vi "Write Micron Configuration.vi"(8 "error in (no error)":errorcluster, 10 "Configuration":T1={"Reference channel"=-1, "Detection Setting IDs"=[130, 130], "Address"="10.0.0.55", "Stream and average"=FALSE}, 11 "Micron Optics Driver in":refnum<class "Micron Optics Driver.lvclass">) -> (0 "error out":errorcluster, 3 "Micron Optics Driver out":refnum<class "Micron Optics Driver.lvclass">)   [LabVIEW 2016, in "Micron Optics Driver.lvclass"]
uses:
  Micron Optics Driver.lvclass
  C:/GitHub/NHMFL_Core/Libraries/Instruments/Instrument Driver/Instrument Driver.lvclass
  Micron optics configuration.ctl
  Instrument Driver/Write User configuration.vi
panel:
  # "CH1\n.\n.\n.\n.\n.\nCH4"
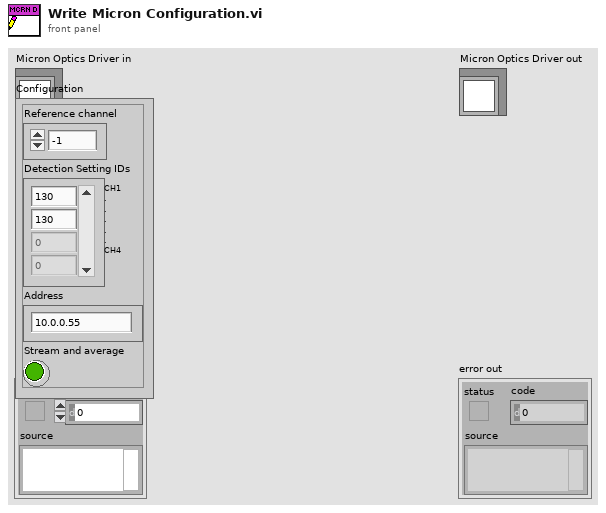
[diagram p1: front panel]
types:
  T1 = typedef "Micron optics configuration.ctl" = cluster{"Reference channel":i32, "Detection Setting IDs":u8[], "Address":string, "Stream and average":bool}
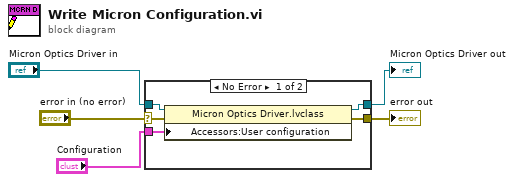
[diagram p0: block diagram]
diagram:
  n1 = case shown="No Error" "error in (no error)" {
    selector: "error in (no error)" -> [w8 w11]
    tunnel: [w7 w11] -> w4
    tunnel: [w9 w12] -> w2
    tunnel: "Micron Optics Driver in" -> [w10 w12]
    tunnel: "Configuration" -> [w6 _]
    frame No Error {
      n2 = property class="Micron Optics Driver.lvclass"(reference=w10, error in=w8, "Accessors:User configuration"=w6) -> (reference out=w9:refnum<class "Micron Optics Driver.lvclass">, error out=w7:errorcluster)
    }
    frame Error {
    }
  }
  "error out" <- w4
  "Micron Optics Driver out" <- w2
